vi "Set Sub Panel.vi"(8 "error in (no error)":errorcluster, 10 "Sub Panel":refnum<vi>, 11 "Contabilidad in":refnum<class "Contabilidad.lvclass">) -> (0 "error out":errorcluster, 3 "Contabilidad out":refnum<class "Contabilidad.lvclass">)   [LabVIEW 2021, in "Contabilidad.lvlib" / "Contabilidad.lvclass"]
uses:
  Contabilidad.lvclass
  Contabilidad.lvclass/Contabilidad.ctl
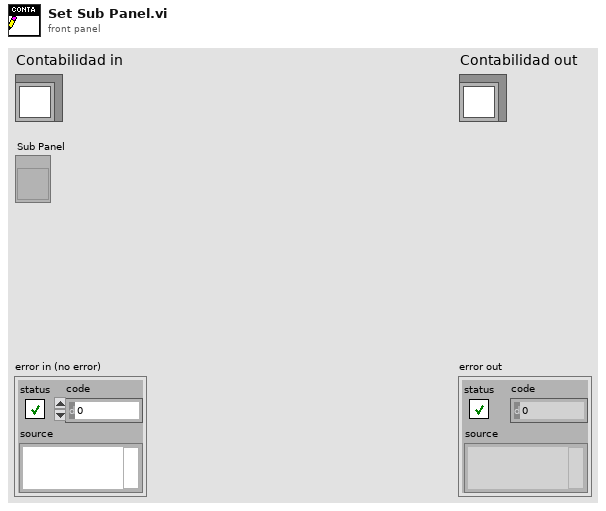
[diagram p1: front panel]
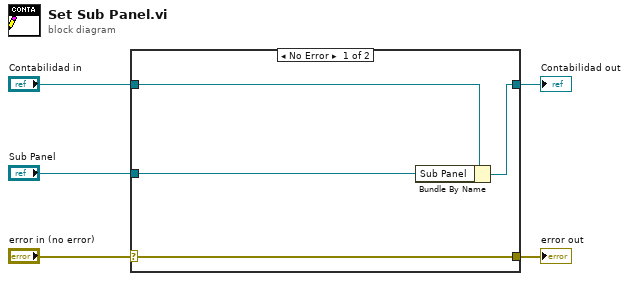
[diagram p0: block diagram]
diagram:
  n1 = case shown="No Error" "error in (no error)" {
    selector: "error in (no error)" -> [w9 w10]
    tunnel: [w9 w10] -> w4
    tunnel: [w7 w11] -> w2
    tunnel: "Contabilidad in" -> [w8 w11]
    tunnel: "Sub Panel" -> [w6 _]
    frame No Error {
      n2 = Bundle By Name(cluster=w8, "Sub Panel"=w6) -> (w7:refnum<class "Contabilidad.lvclass">)
    }
    frame Error {
    }
  }
  "error out" <- w4
  "Contabilidad out" <- w2
